vi "Wrapper-CSM Queue++.vi"(0 "State Queue":string, 1 "Name(\"\" to use uuid)":string, 2 "Response Arguments":string, 7 "Error In (no error)":errorcluster, 9 "Dequeue Timeout(0ms)":i32, 11 "Response Timeout(5000ms)":i32=5000, 12 "Allowed Messages(Empty for all)":string[](array[string])) -> (3 "Name Used":string, 4 "Remaining States":string, 6 "Current State":string, 8 "Arguments":string, 10 ">> Response Source Message >>":T1, 15 ">> Source CSM >>":string)   [LabVIEW 2017]
uses:
  src/user.lib/_NEVSTOP/Communicable State Machine(CSM)/_Support/Typedef/_CSM_Response Source Message.ctl
  src/user.lib/_NEVSTOP/Communicable State Machine(CSM)/Communicable State Machine.lvlib
panel:
  # "Connector Pane"
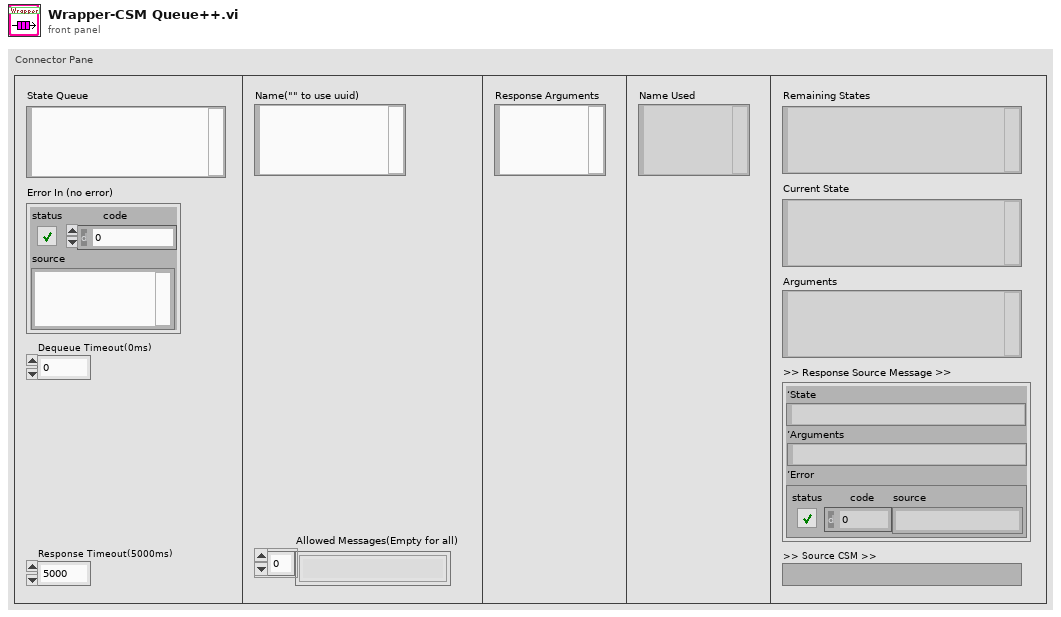
[diagram p1: front panel]
types:
  T1 = typedef "Communicable State Machine.lvlib/_CSM_Response Source Message.ctl" = cluster{"‘State":string, "’Arguments":string, "’Error":errorcluster}
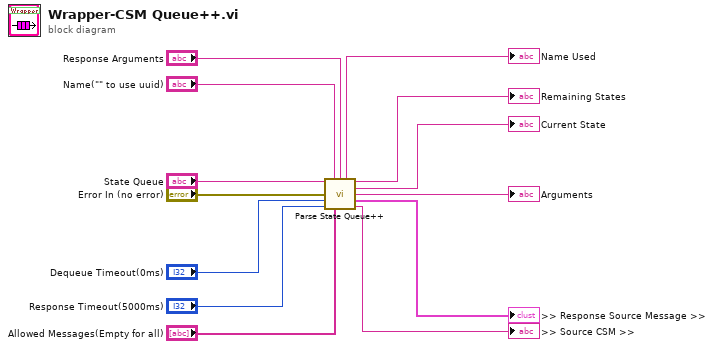
[diagram p0: block diagram]
diagram:
  n1 = call "Parse State Queue++.vi"("State Queue"="State Queue", "Name(\"\" to use uuid)"="Name(\"\" to use uuid)", "Response Arguments"="Response Arguments", "Error In (no error)"="Error In (no error)", "Dequeue Timeout(0ms)"="Dequeue Timeout(0ms)", "Response Timeout(5000ms)"="Response Timeout(5000ms)", "Allowed Messages(Empty for all)"="Allowed Messages(Empty for all)") -> ("Name Used"=→"Name Used":string, "Remaining States"=→"Remaining States":string, "Current State"=→"Current State":string, "Arguments"=→"Arguments":string, ">> Response Source Message >>"=→">> Response Source Message >>":T1, ">> Source CSM >>"=→">> Source CSM >>":string)  [unwired: 3 in]
